vi "MODAQ Configs2Globals v2 RD v1.0.vi"(1 "Configs in":T1={"Watch Circle"={"Set Point Lat (dd)"=0.0, "Set Point Lon (dd)"=0.0, "Yellow Alert Radius (m)"=0.0, "Red Alert Radius (m)"=0.0, "AWOL Radius (m)"=0.0, "Yellow Alert Snooze (min)"=0.0, "Red Alert Snooze (min)"=0.0, "AWOL Radius Snooze (min)"=0.0}, "FTP and AWS"={"AWS Access Key"="", "AWS Secret Key"="", "AWS Bucket"="", "Enable AWS Upload (Summary)"=FALSE, "Enable FTP Upload"=FALSE, "FTP Host"="", "FTP User"="", "FTP Password"="", "Destination write path (pos)"="", "Local file path (pos)"="", "Summary  Upload Interval pos (min)"=0, "Delete Local File After Upload"=FALSE, "Destination write path (pow)"="", "Local file path (pow)"="", "Summary Upload Interval pow (min)"=0, "Enable AWS Upload (TDMS)"=FALSE}, "Email Settings"={"Enable Alerts"=FALSE, "Distribution List (comma separated) 1"="", "Distribution List (comma separated) 2"="", "Sender Email"="", "SMTP"="", "Username"="", "Password"=""}, "Summary File"={"Enable CSV"=FALSE, "CSV Averaging Time (Sec)"=0, "CSV Loop Delay (ms)"=0}, "File Settings"={"Config File Path"="", "Data Folder Path"="", "Raw Mode"="", "Raw Interval (min)"=0, "Raw Sampling Time (min)"=0, "TDMS File Write Interval"=enum."10 Min", "Default Filename"=path "", "Enable TDMS Save (3ph only)"=FALSE}, "Watchdog"={"Watchdog Period (ms)"=0, "Reset System on WD timeout"=FALSE, "Enable RT Watchdog"=FALSE}, "PowGrp0"={"Channel Names"=["", "", "", "", "", "", "", "", "", "", "", ""], "Channel Units"=["", "", "", "", "", "", "", "", "", "", "", ""], "TDMS File Suffix"="", "Channel Datatype"=["", "", "", "", "", "", "", "", "", "", "", ""]}, "Scaling Factors Grp0"=[], "PowGrp0 Sampling"={"PowGrp0 sample rate [Hz]"=5000.0, "PowGrp0 samples per channel"=500}, "Stbd 3 Phase Voltage Scaling"=[50.0, 50.0, 50.0], "Stbd 3 Phase Current Scaling"=[-12.724, -12.739, -12.73]} {"PowGrp0 Sampling"."PowGrp0 sample rate [Hz]" format="%0.2f"; "Watch Circle"."AWOL Radius Snooze (min)" format="%#_13g"; "Watch Circle"."Red Alert Snooze (min)" format="%#_13g"; "Watch Circle"."Yellow Alert Snooze (min)" format="%#_13g"; "Watch Circle"."AWOL Radius (m)" format="%#_13g"; "Watch Circle"."Red Alert Radius (m)" format="%#_13g"; "Watch Circle"."Yellow Alert Radius (m)" format="%#_13g"; "Watch Circle"."Set Point Lon (dd)" format="%#_13g"; "Watch Circle"."Set Point Lat (dd)" format="%#_13g"}, 3 "error in":errorcluster, 4 "Queue in":refnum<queue>) -> (10 "error out":errorcluster)   [LabVIEW 2019]
doc: "Takes the configuration cluster created in Config Load 1 and copies values to global variables. \n\nNOTE: MODAQ makes use of global vairables to propagate configuration constants and other operational data.\n\n2020 NREL"
uses:
  Globals and Definitions/Config Loader TypeDefs/All Tab Controls RDv1.0.ctl
  Globals and Definitions/Config Loader TypeDefs/Watch Circle.ctl
  Globals and Definitions/Config Loader TypeDefs/AWS and FTP.ctl
  Globals and Definitions/Config Loader TypeDefs/Email Settings.ctl
  Globals and Definitions/Config Loader TypeDefs/Summary File.ctl
  Globals and Definitions/Config Loader TypeDefs/File Settings.ctl
  Globals and Definitions/Enum_FileNewInterval.ctl
  Globals and Definitions/Config Loader TypeDefs/Watchdog.ctl
  Globals and Definitions/TDMS Constants.ctl
  Globals and Definitions/System Message.ctl
  Globals and Definitions/Initialization Globals.vi
  Globals and Definitions/TDMS_File_Constants Globals.vi
panel:
  # "PT-EN1-1001"
  # "CT-EN1-1001"
  # "PT-EN1-1002"
  # "CT-EN1-1002"
  # "PT-EN1-1003"
  # "CT-EN1-1003"
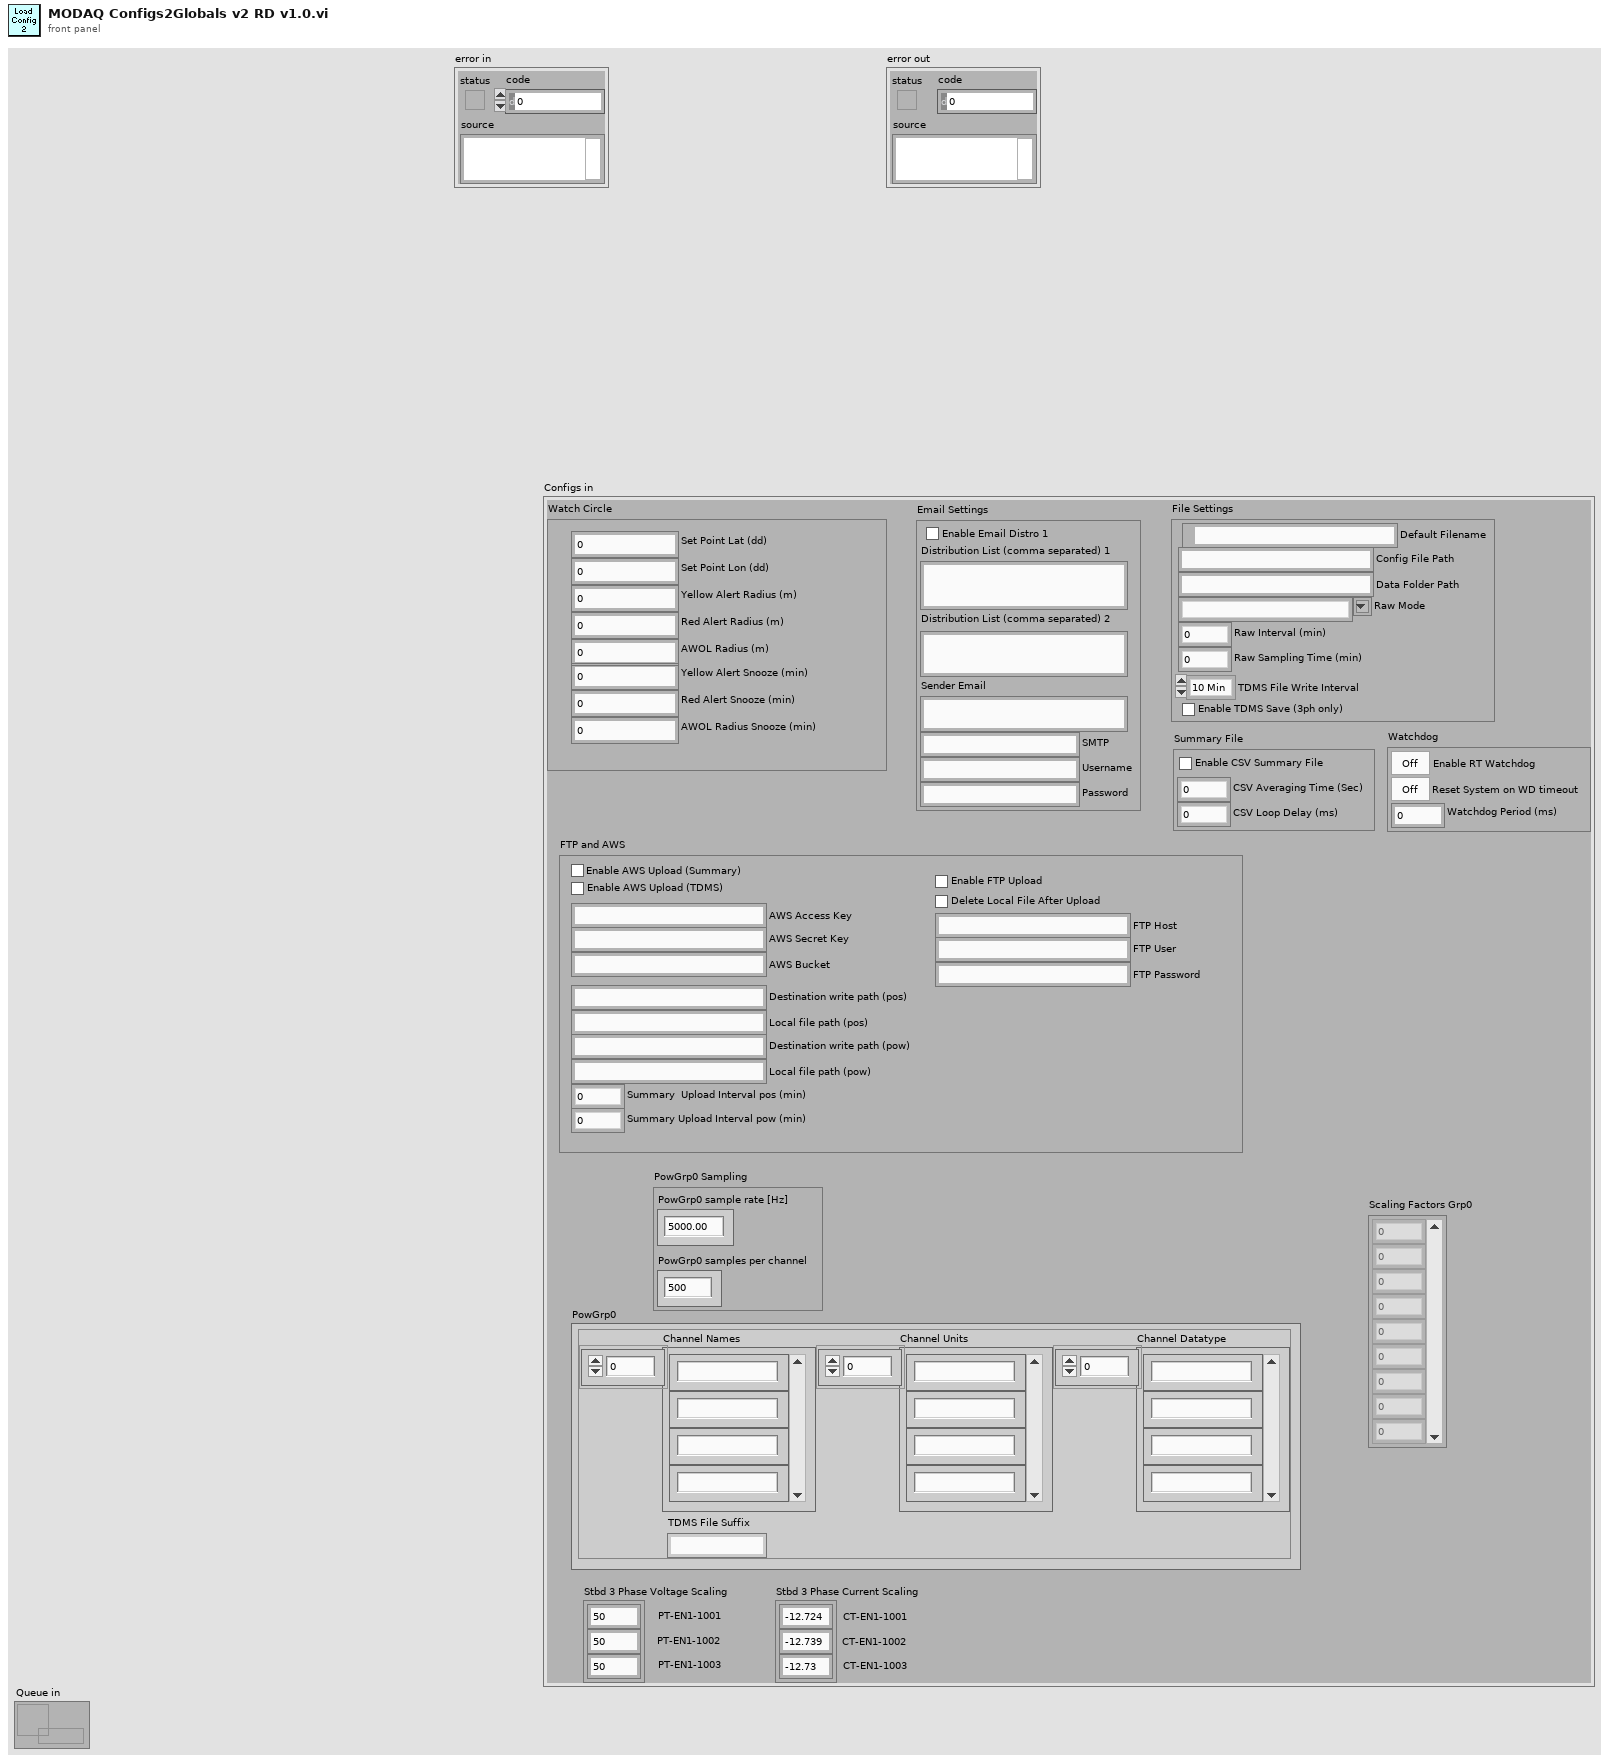
[diagram p1: front panel]
types:
  T1 = typedef "All Tab Controls RDv1.0.ctl" = cluster{"Watch Circle":T2, "FTP and AWS":T3, "Email Settings":T4, "Summary File":T5, "File Settings":T6, "Watchdog":T8, "PowGrp0":T9, "Scaling Factors Grp0":dbl[], "PowGrp0 Sampling":cluster{"PowGrp0 sample rate [Hz]":dbl, "PowGrp0 samples per channel":i32}, "Stbd 3 Phase Voltage Scaling":dbl[], "Stbd 3 Phase Current Scaling":dbl[]}
  T2 = typedef "Watch Circle.ctl" = cluster{"Set Point Lat (dd)":dbl, "Set Point Lon (dd)":dbl, "Yellow Alert Radius (m)":dbl, "Red Alert Radius (m)":dbl, "AWOL Radius (m)":dbl, "Yellow Alert Snooze (min)":dbl, "Red Alert Snooze (min)":dbl, "AWOL Radius Snooze (min)":dbl}
  T3 = typedef "AWS and FTP.ctl" = cluster{"AWS Access Key":string, "AWS Secret Key":string, "AWS Bucket":string, "Enable AWS Upload (Summary)":bool, "Enable FTP Upload":bool, "FTP Host":string, "FTP User":string, "FTP Password":string, "Destination write path (pos)":string, "Local file path (pos)":string, "Summary  Upload Interval pos (min)":i32, "Delete Local File After Upload":bool, "Destination write path (pow)":string, "Local file path (pow)":string, "Summary Upload Interval pow (min)":i32, "Enable AWS Upload (TDMS)":bool}
  T4 = typedef "Email Settings.ctl" = cluster{"Enable Alerts":bool, "Distribution List (comma separated) 1":string, "Distribution List (comma separated) 2":string, "Sender Email":string, "SMTP":string, "Username":string, "Password":string}
  T5 = typedef "Summary File.ctl" = cluster{"Enable CSV":bool, "CSV Averaging Time (Sec)":i32, "CSV Loop Delay (ms)":i32}
  T6 = typedef "File Settings.ctl" = cluster{"Config File Path":string, "Data Folder Path":string, "Raw Mode":string, "Raw Interval (min)":i32, "Raw Sampling Time (min)":i32, "TDMS File Write Interval":T7, "Default Filename":path, "Enable TDMS Save (3ph only)":bool}
  T7 = typedef "Enum_FileNewInterval.ctl" = enum16{"10 Min", "Hourly", "Daily", "Weekly", "Monthly"}
  T8 = typedef "Watchdog.ctl" = cluster{"Watchdog Period (ms)":u32, "Reset System on WD timeout":bool, "Enable RT Watchdog":bool}
  T9 = typedef "TDMS Constants.ctl" = cluster{"Channel Names":string[], "Channel Units":string[], "TDMS File Suffix":string, "Channel Datatype":string[]}
  T10 = cluster{"PowGrp0 sample rate [Hz]":dbl, "PowGrp0 samples per channel":i32}
  T11 = typedef "System Message.ctl" = cluster{"Message Tag":string, "Message Body":string, "Snooze Time (s)":dbl, "Snooze Alert?":bool, "Log Event?":bool, "Send Email":i32}
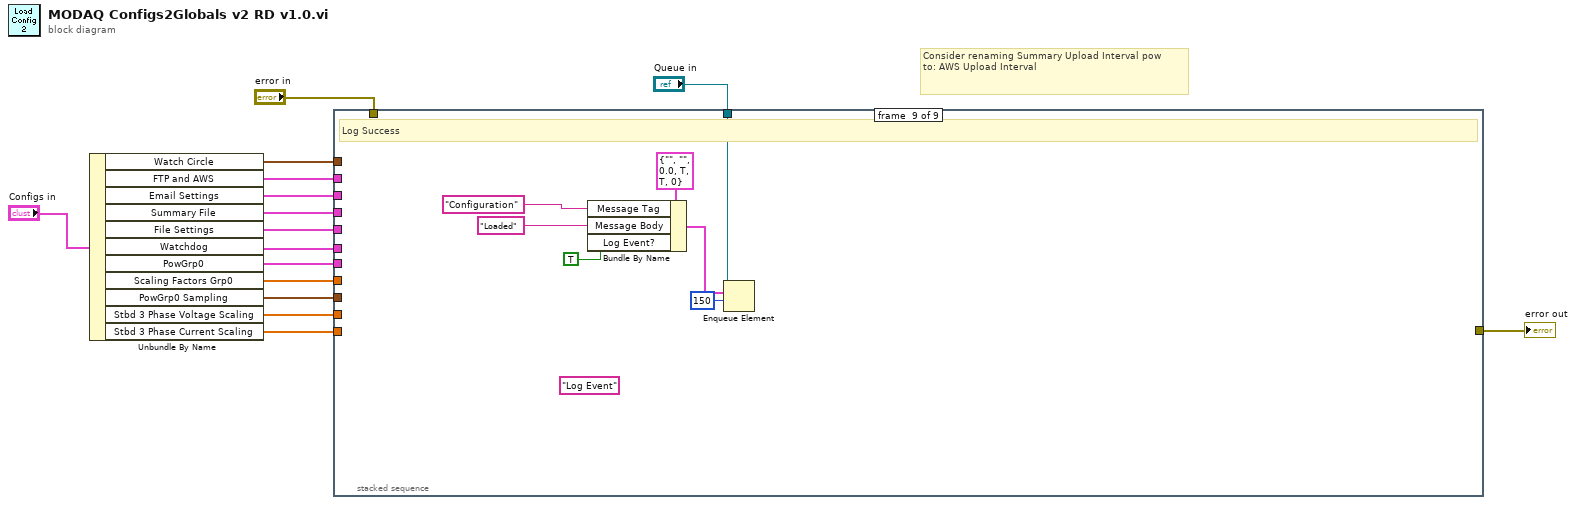
[diagram p0: block diagram]
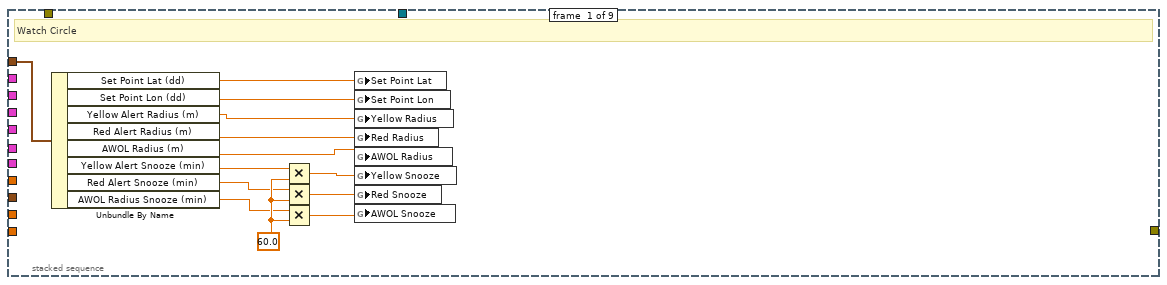
[diagram p2: hidden frame]
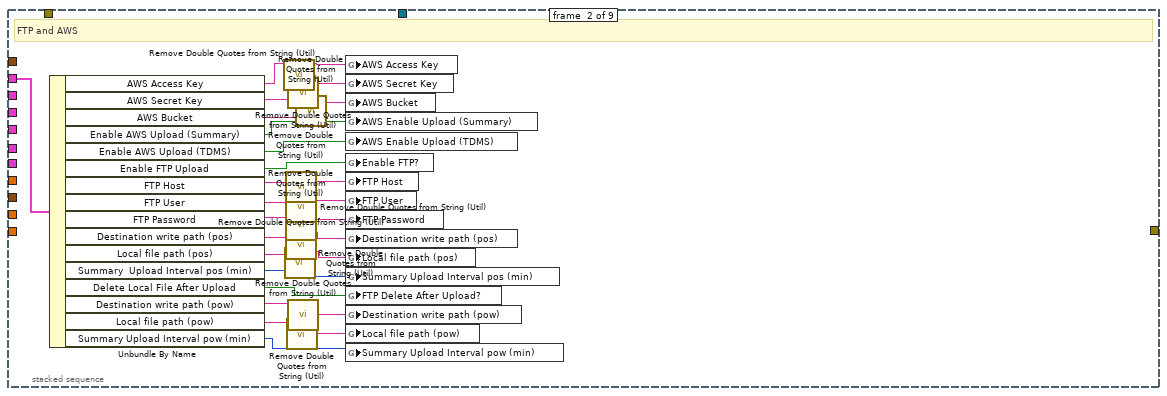
[diagram p3: hidden frame]
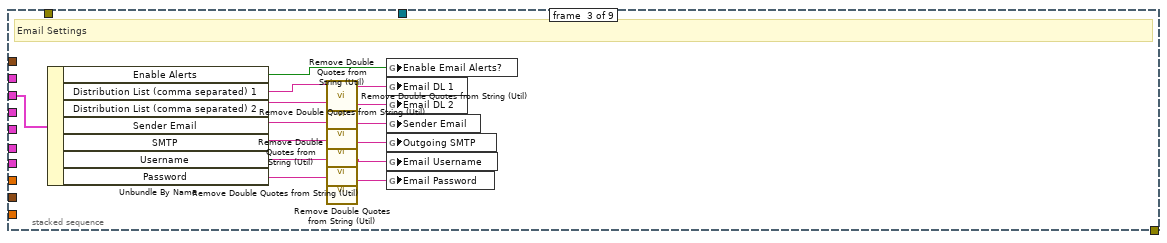
[diagram p4: hidden frame]
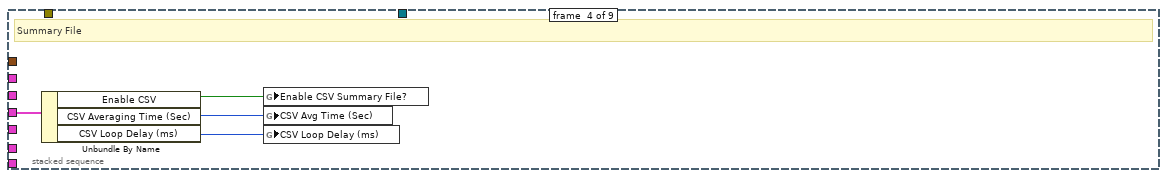
[diagram p5: hidden frame]
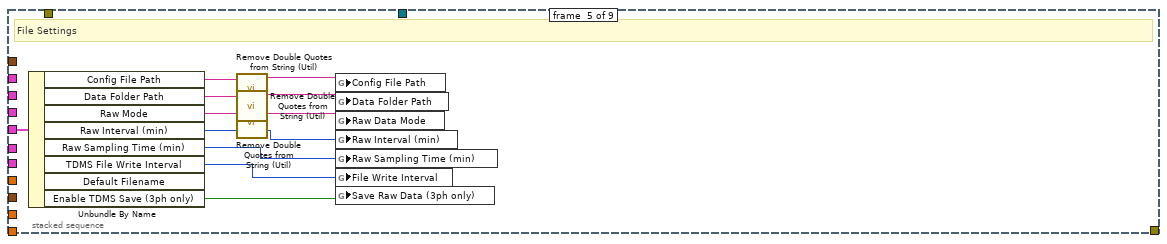
[diagram p6: hidden frame]
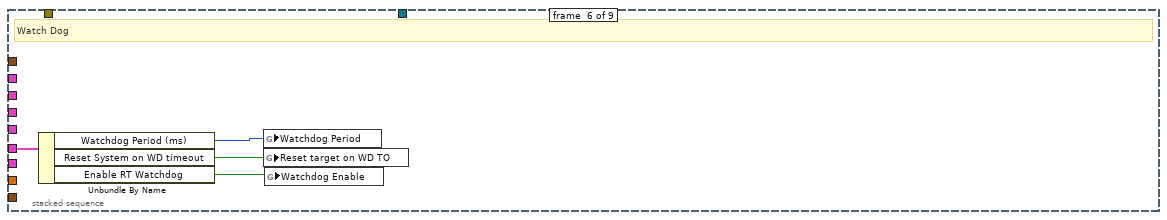
[diagram p7: hidden frame]
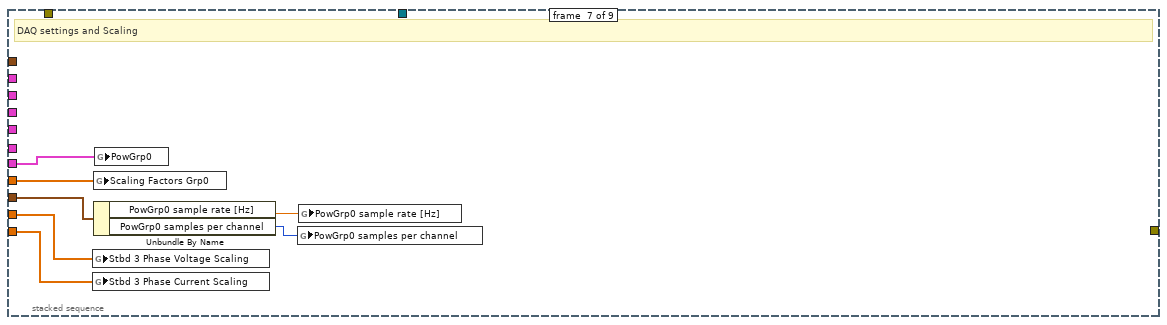
[diagram p8: hidden frame]
diagram:
  # "Consider renaming Summary Upload Interval pow\nto: AWS Upload Interval"
  n1 = Unbundle By Name("Configs in") -> ("Watch Circle"=w14:T2, "FTP and AWS"=w13:T3, "Email Settings"=w12:T4, "Summary File"=w11:T5, "File Settings"=w10:T6, "Watchdog"=w9:T8, "PowGrp0"=w8:T9, "Scaling Factors Grp0"=w7:dbl[], "PowGrp0 Sampling"=w6:T10, "Stbd 3 Phase Voltage Scaling"=w5:dbl[], "Stbd 3 Phase Current Scaling"=w4:dbl[])
  n2 = stacked-sequence {
    tunnel: w14 -> [w28 _ _ _ _ _ _ _ _]
    tunnel: w13 -> [_ w29 _ _ _ _ _ _ _]
    tunnel: w12 -> [_ _ w69 _ _ _ _ _ _]
    tunnel: w11 -> [_ _ _ w73 _ _ _ _ _]
    tunnel: w10 -> [_ _ _ _ w84 _ _ _ _]
    tunnel: w9 -> [_ _ _ _ _ w88 _ _ _]
    tunnel: w8 -> [_ _ _ _ _ _ w95 _ _]
    tunnel: w7 -> [_ _ _ _ _ _ w91 _ _]
    tunnel: w6 -> [_ _ _ _ _ _ w94 _ _]
    tunnel: w5 -> [_ _ _ _ _ _ w90 _ _]
    tunnel: w4 -> [_ _ _ _ _ _ w89 _ _]
    tunnel: "Queue in" -> [_ _ _ _ _ _ _ _ w98]
    tunnel: "error in" -> [_ _ _ _ _ _ _ w96 _]
    tunnel: [_ _ _ _ _ _ _ w96 _] -> w1
    frame #0 {
      w27 = 60.0 ("y")
      # "Watch Circle"
      n3 = Unbundle By Name(w28) -> ("Set Point Lat (dd)"=w23:dbl, "Set Point Lon (dd)"=w22:dbl, "Yellow Alert Radius (m)"=w21:dbl, "Red Alert Radius (m)"=w20:dbl, "AWOL Radius (m)"=w19:dbl, "Yellow Alert Snooze (min)"=w26:dbl, "Red Alert Snooze (min)"=w25:dbl, "AWOL Radius Snooze (min)"=w24:dbl)
      n4 = Multiply(x=w26, y=w27) -> (x*y=w18:dbl)
      n5 = Multiply(x=w25, y=w27) -> (x*y=w17:dbl)
      n6 = Multiply(x=w24, y=w27) -> (x*y=w16:dbl)
      n7 = global write "Initialization Globals.vi" "Set Point Lat"(w23) -> ()
      n8 = global write "Initialization Globals.vi" "Set Point Lon"(w22) -> ()
      n9 = global write "Initialization Globals.vi" "Yellow Radius"(w21) -> ()
      n10 = global write "Initialization Globals.vi" "Red Radius"(w20) -> ()
      n11 = global write "Initialization Globals.vi" "AWOL Radius"(w19) -> ()
      n12 = global write "Initialization Globals.vi" "Yellow Snooze"(w18) -> ()
      n13 = global write "Initialization Globals.vi" "Red Snooze"(w17) -> ()
      n14 = global write "Initialization Globals.vi" "AWOL Snooze"(w16) -> ()
    }
    frame #1 {
      # "FTP and AWS"
      n15 = Unbundle By Name(w29) -> ("AWS Access Key"=w50:string, "AWS Secret Key"=w48:string, "AWS Bucket"=w46:string, "Enable AWS Upload (Summary)"=w55:bool, "Enable AWS Upload (TDMS)"=w31:bool, "Enable FTP Upload"=w30:bool, "FTP Host"=w44:string, "FTP User"=w42:string, "FTP Password"=w40:string, "Destination write path (pos)"=w38:string, "Local file path (pos)"=w36:string, "Summary  Upload Interval pos (min)"=w54:i32, "Delete Local File After Upload"=w53:bool, "Destination write path (pow)"=w34:string, "Local file path (pow)"=w32:string, "Summary Upload Interval pow (min)"=w52:i32)
      n16 = call "Remove Double Quotes from String (Util).vi"("String In"=w50) -> ("Quotes Removed"=w51:string)  [unwired: 10 in]
      n17 = call "Remove Double Quotes from String (Util).vi"("String In"=w36) -> ("Quotes Removed"=w37:string)  [unwired: 10 in]
      n18 = call "Remove Double Quotes from String (Util).vi"("String In"=w44) -> ("Quotes Removed"=w45:string)  [unwired: 10 in]
      n19 = call "Remove Double Quotes from String (Util).vi"("String In"=w42) -> ("Quotes Removed"=w43:string)  [unwired: 10 in]
      n20 = call "Remove Double Quotes from String (Util).vi"("String In"=w40) -> ("Quotes Removed"=w41:string)  [unwired: 10 in]
      n21 = call "Remove Double Quotes from String (Util).vi"("String In"=w38) -> ("Quotes Removed"=w39:string)  [unwired: 10 in]
      n22 = call "Remove Double Quotes from String (Util).vi"("String In"=w32) -> ("Quotes Removed"=w33:string)  [unwired: 10 in]
      n23 = call "Remove Double Quotes from String (Util).vi"("String In"=w48) -> ("Quotes Removed"=w49:string)  [unwired: 10 in]
      n24 = call "Remove Double Quotes from String (Util).vi"("String In"=w34) -> ("Quotes Removed"=w35:string)  [unwired: 10 in]
      n25 = call "Remove Double Quotes from String (Util).vi"("String In"=w46) -> ("Quotes Removed"=w47:string)  [unwired: 10 in]
      n26 = global write "Initialization Globals.vi" "AWS Access Key"(w51) -> ()
      n27 = global write "Initialization Globals.vi" "AWS Secret Key"(w49) -> ()
      n28 = global write "Initialization Globals.vi" "AWS Bucket"(w47) -> ()
      n29 = global write "Initialization Globals.vi" "AWS Enable Upload (Summary)"(w55) -> ()
      n30 = global write "Initialization Globals.vi" "AWS Enable Upload (TDMS)"(w31) -> ()
      n31 = global write "Initialization Globals.vi" "Enable FTP?"(w30) -> ()
      n32 = global write "Initialization Globals.vi" "FTP Host"(w45) -> ()
      n33 = global write "Initialization Globals.vi" "FTP User"(w43) -> ()
      n34 = global write "Initialization Globals.vi" "FTP Password"(w41) -> ()
      n35 = global write "Initialization Globals.vi" "Destination write path (pos)"(w39) -> ()
      n36 = global write "Initialization Globals.vi" "Local file path (pos)"(w37) -> ()
      n37 = global write "Initialization Globals.vi" "Summary Upload Interval pos (min)"(w54) -> ()
      n38 = global write "Initialization Globals.vi" "FTP Delete After Upload?"(w53) -> ()
      n39 = global write "Initialization Globals.vi" "Destination write path (pow)"(w35) -> ()
      n40 = global write "Initialization Globals.vi" "Local file path (pow)"(w33) -> ()
      n41 = global write "Initialization Globals.vi" "Summary Upload Interval pow (min)"(w52) -> ()
    }
    frame #2 {
      # "Email Settings"
      n42 = Unbundle By Name(w69) -> ("Enable Alerts"=w68:bool, "Distribution List (comma separated) 1"=w56:string, "Distribution List (comma separated) 2"=w58:string, "Sender Email"=w60:string, "SMTP"=w62:string, "Username"=w64:string, "Password"=w66:string)
      n43 = call "Remove Double Quotes from String (Util).vi"("String In"=w56) -> ("Quotes Removed"=w57:string)  [unwired: 10 in]
      n44 = call "Remove Double Quotes from String (Util).vi"("String In"=w58) -> ("Quotes Removed"=w59:string)  [unwired: 10 in]
      n45 = call "Remove Double Quotes from String (Util).vi"("String In"=w60) -> ("Quotes Removed"=w61:string)  [unwired: 10 in]
      n46 = call "Remove Double Quotes from String (Util).vi"("String In"=w62) -> ("Quotes Removed"=w63:string)  [unwired: 10 in]
      n47 = call "Remove Double Quotes from String (Util).vi"("String In"=w64) -> ("Quotes Removed"=w65:string)  [unwired: 10 in]
      n48 = call "Remove Double Quotes from String (Util).vi"("String In"=w66) -> ("Quotes Removed"=w67:string)  [unwired: 10 in]
      n49 = global write "Initialization Globals.vi" "Enable Email Alerts?"(w68) -> ()
      n50 = global write "Initialization Globals.vi" "Email DL 1"(w57) -> ()
      n51 = global write "Initialization Globals.vi" "Email DL 2"(w59) -> ()
      n52 = global write "Initialization Globals.vi" "Sender Email"(w61) -> ()
      n53 = global write "Initialization Globals.vi" "Outgoing SMTP"(w63) -> ()
      n54 = global write "Initialization Globals.vi" "Email Username"(w65) -> ()
      n55 = global write "Initialization Globals.vi" "Email Password"(w67) -> ()
    }
    frame #3 {
      # "Summary File"
      n56 = Unbundle By Name(w73) -> ("Enable CSV"=w71:bool, "CSV Averaging Time (Sec)"=w72:i32, "CSV Loop Delay (ms)"=w70:i32)
      n57 = global write "Initialization Globals.vi" "Enable CSV Summary File?"(w71) -> ()
      n58 = global write "Initialization Globals.vi" "CSV Avg Time (Sec)"(w72) -> ()
      n59 = global write "Initialization Globals.vi" "CSV Loop Delay (ms)"(w70) -> ()
    }
    frame #4 {
      # "File Settings"
      n60 = Unbundle By Name(w84) -> ("Config File Path"=w83:string, "Data Folder Path"=w81:string, "Raw Mode"=w79:string, "Raw Interval (min)"=w76:i32, "Raw Sampling Time (min)"=w77:i32, "TDMS File Write Interval"=w75:T7, "Enable TDMS Save (3ph only)"=w74:bool)  [unwired: 1 out]
      n61 = call "Remove Double Quotes from String (Util).vi"("String In"=w83) -> ("Quotes Removed"=w82:string)  [unwired: 10 in]
      n62 = call "Remove Double Quotes from String (Util).vi"("String In"=w81) -> ("Quotes Removed"=w80:string)  [unwired: 10 in]
      n63 = call "Remove Double Quotes from String (Util).vi"("String In"=w79) -> ("Quotes Removed"=w78:string)  [unwired: 10 in]
      n64 = global write "Initialization Globals.vi" "Config File Path"(w82) -> ()
      n65 = global write "Initialization Globals.vi" "Data Folder Path"(w80) -> ()
      n66 = global write "Initialization Globals.vi" "Raw Data Mode"(w78) -> ()
      n67 = global write "Initialization Globals.vi" "Raw Interval (min)"(w76) -> ()
      n68 = global write "Initialization Globals.vi" "Raw Sampling Time (min)"(w77) -> ()
      n69 = global write "Initialization Globals.vi" "File Write Interval"(w75) -> ()
      n70 = global write "Initialization Globals.vi" "Save Raw Data (3ph only)"(w74) -> ()
    }
    frame #5 {
      # "Watch Dog"
      n71 = Unbundle By Name(w88) -> ("Watchdog Period (ms)"=w87:u32, "Reset System on WD timeout"=w86:bool, "Enable RT Watchdog"=w85:bool)
      n72 = global write "Initialization Globals.vi" "Watchdog Period"(w87) -> ()
      n73 = global write "Initialization Globals.vi" "Reset target on WD TO"(w86) -> ()
      n74 = global write "Initialization Globals.vi" "Watchdog Enable"(w85) -> ()
    }
    frame #6 {
      # "DAQ settings and Scaling"
      n75 = global write "Initialization Globals.vi" "Stbd 3 Phase Voltage Scaling"(w90) -> ()
      n76 = global write "Initialization Globals.vi" "Stbd 3 Phase Current Scaling"(w89) -> ()
      n77 = global write "Initialization Globals.vi" "Scaling Factors Grp0"(w91) -> ()
      n78 = Unbundle By Name(w94) -> ("PowGrp0 sample rate [Hz]"=w93:dbl, "PowGrp0 samples per channel"=w92:i32)
      n79 = global write "TDMS_File_Constants Globals.vi" "PowGrp0"(w95) -> ()
      n80 = global write "Initialization Globals.vi" "PowGrp0 samples per channel"(w92) -> ()
      n81 = global write "Initialization Globals.vi" "PowGrp0 sample rate [Hz]"(w93) -> ()
    }
    frame #7 {
    }
    frame #8 {
      (unwired) "Log Event" ("Message Tag")
      # "Log Success"
      n82 = Bundle By Name(cluster=T11 {"Message Tag"="", "Message Body"="", "Snooze Time (s)"=0.0, "Snooze Alert?"=TRUE, "Log Event?"=TRUE, "Send Email"=0}, "Message Tag"="Configuration", "Message Body"="Loaded", "Log Event?"=TRUE) -> (w99:T11)
      n83 = Enqueue Element(queue=w98, element=w99, timeout in ms (-1)=150) -> ()  [unwired: 1 in, 3 out]
    }
  }
  "error out" <- w1
